vi "_Cluster AutoSizing Core SubVI.vi"(6 "recursive":bool, 8 "error in (no error)":errorcluster, 9 "type":T1(ring), 10 "QD Launch VI Panel?":bool, 11 "VI in":refnum<vi>) -> (0 "error out":errorcluster, 2 "Changed?":bool, 3 "VI out":refnum<vi>)   [LabVIEW 2017, in "Cluster AutoSizing.lvlib"]
uses:
  Cluster AutoSizing.lvlib
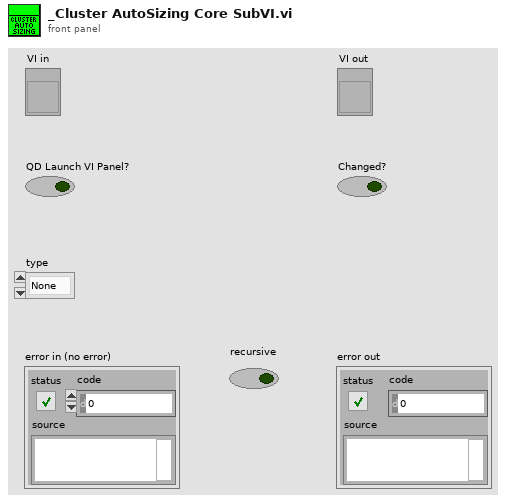
[diagram p1: front panel]
types:
  T1 = enum16{"None", "Size to Fit", "Arrange Horizontally", "Arrange Veritcally"}
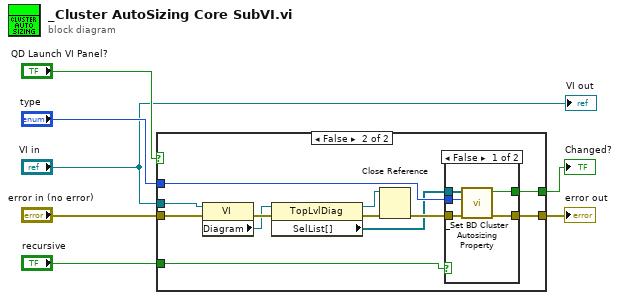
[diagram p0: block diagram]
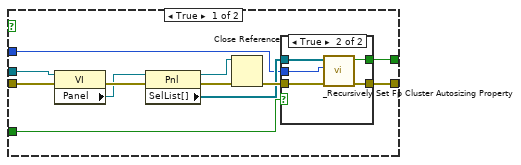
[diagram p2: hidden frame]
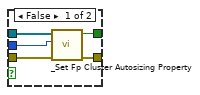
[diagram p3: hidden frame]
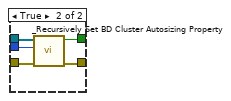
[diagram p4: hidden frame]
diagram:
  n1 = case shown="False" "QD Launch VI Panel?" {
    tunnel: "error in (no error)" -> [w19 w41]
    tunnel: [w11 w33] -> w5
    tunnel: "VI in" -> [w17 w39]
    tunnel: [w16 w38] -> w6
    tunnel: "type" -> [w9 w32]
    tunnel: "recursive" -> [w8 w30]
    frame True {
      n2 = property class="VI"(reference=w17, error in=w19) -> (error out=w15:errorcluster, "Panel"=w14:refnum<vi>)  [unwired: 1 out]
      n3 = property class="Pnl"(reference=w14, error in=w15) -> (reference out=w12:refnum<vi>, error out=w13:errorcluster, "SelList[]"=w10:refnum<vi>[])
      n4 = Close Reference(reference=w12, error in (no error)=w13) -> (error out=w18:errorcluster)
      n5 = case shown="True" w8 {
        tunnel: w18 -> [w24 w28]
        tunnel: [w23 w26] -> w16
        tunnel: [w22 w25] -> w11
        tunnel: w10 -> [w21 w29]
        tunnel: w9 -> [w20 w27]
        frame False {
          n6 = call "_Set Fp Cluster Autosizing Property.vi"("error in (no error)"=w24, "type"=w20, "SelList[]"=w21) -> ("error out"=w22:errorcluster, "Changed"=w23:bool)  [unwired: 7 in]
        }
        frame True {
          n7 = call "_Recursively Set Fp Cluster Autosizing Property.vi"("error in (no error)"=w28, "type"=w27, "SelList[]"=w29) -> ("error out"=w25:errorcluster, "Changed"=w26:bool)  [unwired: 7 in]
        }
      }
    }
    frame False {
      n8 = property class="VI"(reference=w39, error in=w41) -> (error out=w37:errorcluster, "Diagram"=w36:refnum<vi>)  [unwired: 1 out]
      n9 = property class="TopLvlDiag"(reference=w36, error in=w37) -> (reference out=w34:refnum<vi>, error out=w35:errorcluster, "SelList[]"=w31:refnum<vi>[])
      n10 = Close Reference(reference=w34, error in (no error)=w35) -> (error out=w40:errorcluster)
      n11 = case shown="False" w30 {
        tunnel: w40 -> [w46 w51]
        tunnel: [w45 w47] -> w38
        tunnel: [w44 w48] -> w33
        tunnel: w32 -> [w43 w50]
        tunnel: w31 -> [w42 w49]
        frame False {
          n12 = call "_Set BD Cluster Autosizing Property.vi"("error in (no error)"=w46, "type"=w43, "SelList[]"=w42) -> ("error out"=w44:errorcluster, "changed"=w45:bool)  [unwired: 7 in]
        }
        frame True {
          n13 = call "_Recursively Set BD Cluster Autosizing Property.vi"("error in (no error)"=w51, "type"=w50, "SelList[]"=w49) -> ("error out"=w48:errorcluster, "changed?"=w47:bool)  [unwired: 7 in]
        }
      }
    }
  }
  "Changed?" <- w6
  "error out" <- w5
  "VI out" <- "VI in"
